vi "Configure Dialog.vi"(8 "error in (no error)":errorcluster, 11 "Configure Start Trigger [STT] Msg.lvclass":refnum<class "Configure Start Trigger [STT] Msg.lvclass">) -> (0 "error out":errorcluster, 2 "Ok?":bool, 3 "Configure Start Trigger [STT] Msg.lvclass":refnum<class "Configure Start Trigger [STT] Msg.lvclass">)   [LabVIEW 2015, in "CS++Fgen.lvlib" / "Configure Start Trigger [STT] Msg.lvclass"]
uses:
  Configure Start Trigger [STT] Msg.lvclass
  Configure Start Trigger [STT] Msg.lvclass/Configure Start Trigger [STT] Msg.ctl
panel:
  in  "Trigger Slope":i32
  in  "Trigger Source":string
  in  "Channel Name":string
  in  "Cancel Button":bool
  in  "OK Button":bool
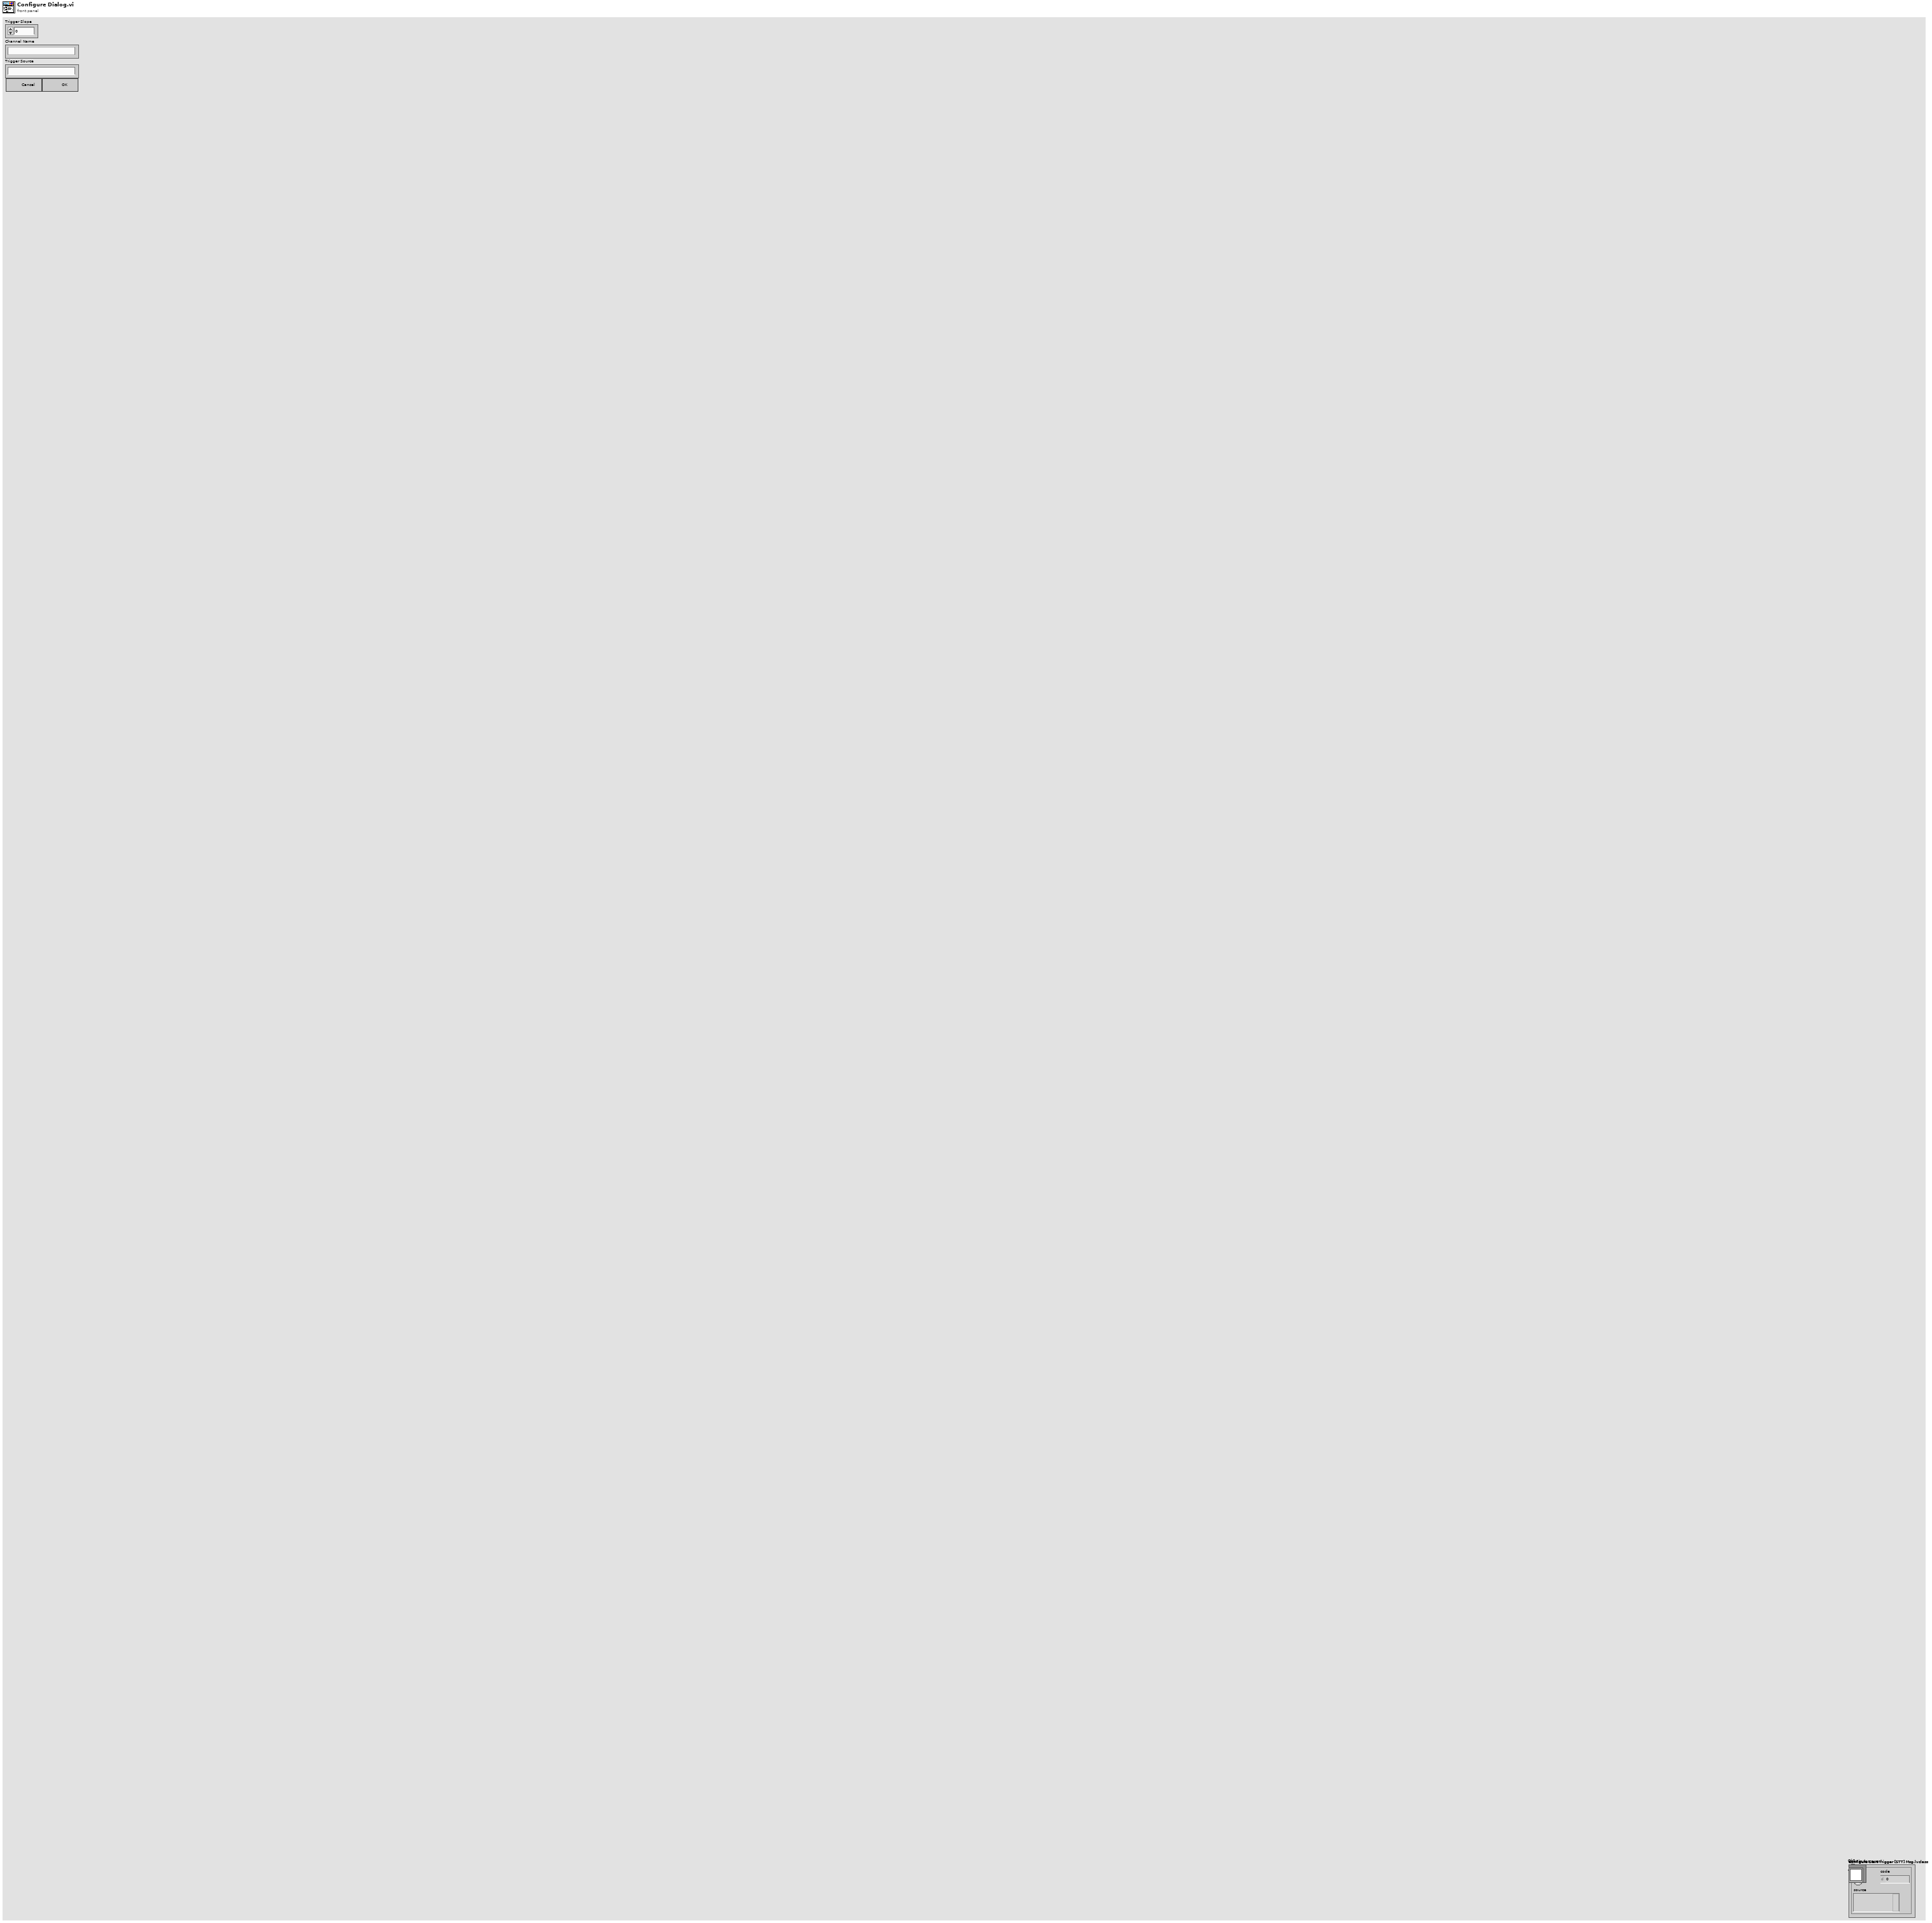
[diagram p1: front panel]
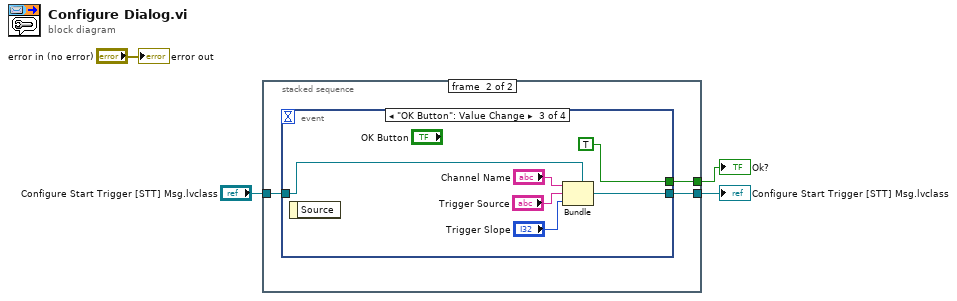
[diagram p0: block diagram]
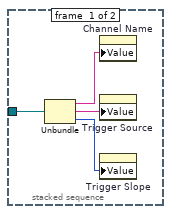
[diagram p2: hidden frame]
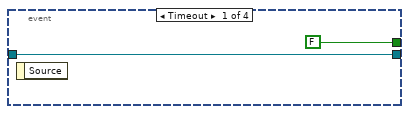
[diagram p3: hidden frame]
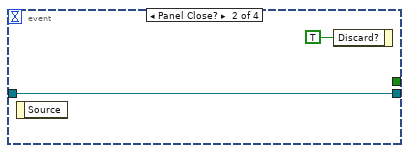
[diagram p4: hidden frame]
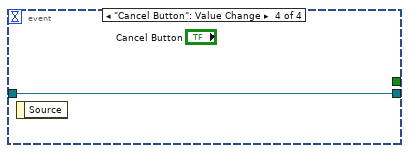
[diagram p5: hidden frame]
diagram:
  n1 = stacked-sequence {
    tunnel: [_ w11] -> w3
    tunnel: [_ w10] -> w2
    tunnel: "Configure Start Trigger [STT] Msg.lvclass" -> [w8 w9]
    frame #0 {
      n2 = Unbundle ("Seq0Unbundler")(w8) -> (w7:string, w6:string, w5:i32)
      n3 = property on="Channel Name" class="Str"("Value"=w7) -> ()  [unwired: 2 in, 2 out]
      n4 = property on="Trigger Source" class="Str"("Value"=w6) -> ()  [unwired: 2 in, 2 out]
      n5 = property on="Trigger Slope" class="DigNum (strict)"("Value"=w5) -> ()  [unwired: 2 in, 2 out]
    }
    frame #1 {
      n6 = event shown="[2] \"OK Button\": Value Change" {
        selector: _ -> [_ _ _ _]
        dyn-events: _ -> [_ _ _ _]
        timeout: _ -> [_ _ _ _]
        tunnel: [w12 w14 w19 w22] -> w10
        tunnel: w9 -> [w12 w14 w21 w22]
        tunnel: [FALSE _ TRUE _] -> w11
        event Timeout {
          n7 = event-data() -> ()  [unwired: 1 in, 1 out]
        }
        event Panel Close? {
          n8 = event-data() -> ()  [unwired: 1 in, 1 out]
          n9 = event-data ("Event Filter Node")("Discard?"=TRUE) -> ()  [unwired: 1 in, 1 out]
        }
        event "OK Button": Value Change {
          n10 = event-data() -> ()  [unwired: 1 in, 1 out]
          n11 = Bundle ("Main-Bundler")(cluster=w21, "Channel Name", "Trigger Source", "Trigger Slope") -> (w19:refnum<class "Configure Start Trigger [STT] Msg.lvclass">)
        }
        event "Cancel Button": Value Change {
          n12 = event-data() -> ()  [unwired: 1 in, 1 out]
        }
      }
    }
  }
  "Ok?" <- w3
  "Configure Start Trigger [STT] Msg.lvclass" <- w2
  "error out" <- "error in (no error)"
